vi "OFDMRX.vi"(0 "received waveform":T1 {"Y" format="%.3f"; "dt" format="%^.2e"; "t0" format="%.4f"}, 1 "Frequency Offset":dbl, 2 "Channel Taps":dbl[](array[numeric]), 3 "Equalize":bool, 4 "Transmitter Properties":T2 {"Window" items=["Rectangular", "Bohman", "Parzen", "Bartlett-Hanning", "Blackman-Nuttall", "Blackman", "Hanning", "Hamming", "Welch", "Exact Blackman", "Blackman-Harris", "Triangle"]}) -> (5 "Output Bits":bool[](array[boolean]))   [LabVIEW 2020]
doc: "This sub-VI encompasses all of the receiver sub-VIs. Note that frequency offset and channel taps need not be specified if no correction is desired or needed.\n\nFor more information about the operation of the individual modules, see their respective descriptions and comments."
uses:
  <vilib>/addons/Modulation/Analog/controls/Complex Data Waveform.ctl
  <vilib>/addons/Modulation/niAMT.lvlib
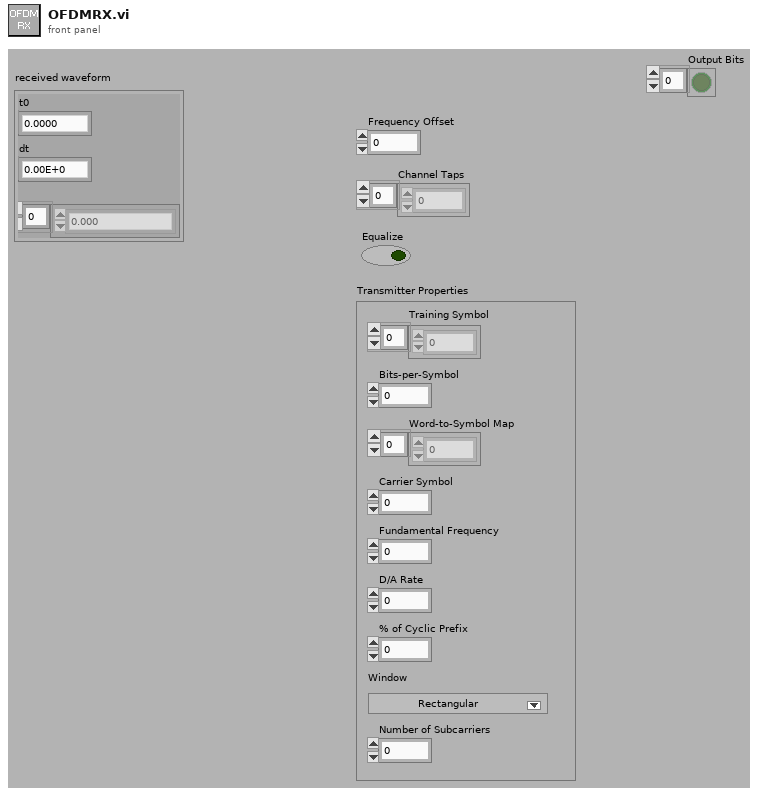
[diagram p1: front panel]
types:
  T1 = typedef "niAMT.lvlib/Complex Data Waveform.ctl" = cluster{"t0":dbl, "dt":dbl, "Y":cdb[]}
  T2 = cluster{"Word-to-Symbol Map":cdb[], "% of Cyclic Prefix":dbl, "Training Symbol":cdb[], "Bits-per-Symbol":i32, "Carrier Symbol":cdb, "Fundamental Frequency":dbl, "D/A Rate":dbl, "Window":u16, "Number of Subcarriers":i32}
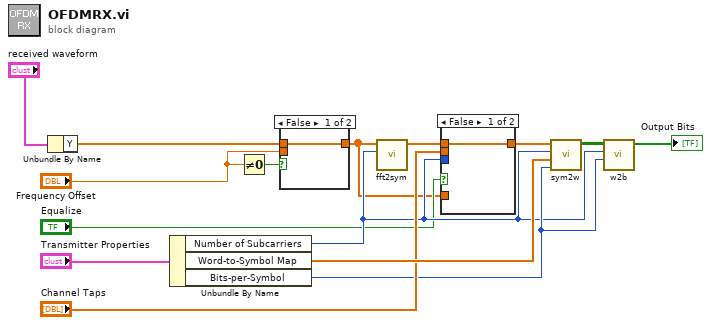
[diagram p0: block diagram]
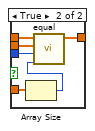
[diagram p2: hidden frame]
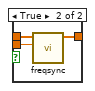
[diagram p3: hidden frame]
diagram:
  n1 = Unbundle By Name("received waveform") -> ("Y"=w1:cdb[])
  n2 = Unbundle By Name("Transmitter Properties") -> ("Number of Subcarriers"=w7:i32, "Word-to-Symbol Map"=w12:cdb[], "Bits-per-Symbol"=w8:i32)
  n3 = Not Equal To 0?(x="Frequency Offset") -> (x != 0?=w6:bool)
  n4 = case shown="False" w6 {
    tunnel: w1 -> [w16 w19]
    tunnel: "Frequency Offset" -> [_ w18]
    tunnel: [w16 w17] -> w3
    frame False {
    }
    frame True {
      n5 = call "freqsync.vi"("Frequency Offset"=w18, "Offset Signal"=w19) -> ("Corrected Signal"=w17:cdb[])  [unwired: 9 in]
    }
  }
  n6 = call "fft2sym.vi"("Number of Subcarriers"=w7, "Time Domain In"=w3) -> ("Parallel Symbol Out"=w11:cdb[])  [unwired: 6 in]
  n7 = case shown="False" "Equalize" {
    tunnel: w11 -> [w20 w26]
    tunnel: [w20 w25] -> w10
    tunnel: "Channel Taps" -> [_ w24]
    tunnel: w7 -> [_ w23]
    tunnel: w3 -> [_ w22]
    frame False {
    }
    frame True {
      n8 = Array Size(array=w22) -> (size(s)=w21:i32)
      n9 = call "equal.vi"("Symbol Size"=w21, "Number of Subcarriers"=w23, "Channel Taps"=w24, "Unequalized Signal"=w26) -> ("Equalized Signal"=w25:cdb[])  [unwired: 7 in]
    }
  }
  n10 = call "sym2w.vi"("Bits-per-Symbol"=w8, "Word-to-Symbol Map"=w12, "Number of Subcarriers"=w7, "Parallel Symbol Input"=w10) -> ("Parallel Word Output"=w15:bool[][])  [unwired: 7 in]
  n11 = call "w2b.vi"("Bits-per-Symbol"=w8, "Number of Subcarriers"=w7, "Parallel Word In"=w15) -> ("Parallel Output"=→"Output Bits":bool[])  [unwired: 8 in]
